vi "S2C_ExeScriptResultCalc.vi"(8 "Error In":errorcluster, 11 "Measurement":string) -> (0 "Error Out":errorcluster, 1 "LastMeas?":bool, 2 "Result":T1, 3 "Data":string[][](array[string]))   [LabVIEW 2015]
doc: "Determines the result for the currently executing line item, and updates the measurement and result in the data array."
uses:
  Controls/S2C_ResultStatus.ctl
  Globals/S2C_Globals.vi
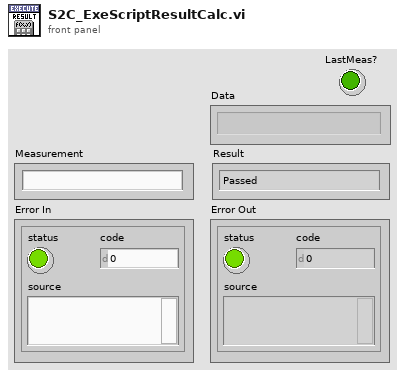
[diagram p1: front panel]
types:
  T1 = typedef "S2C_ResultStatus.ctl" = enum16{"Passed", "Failed", "Logged", "Aborted", "Error", "Testing...", "Paused", "No Record"}
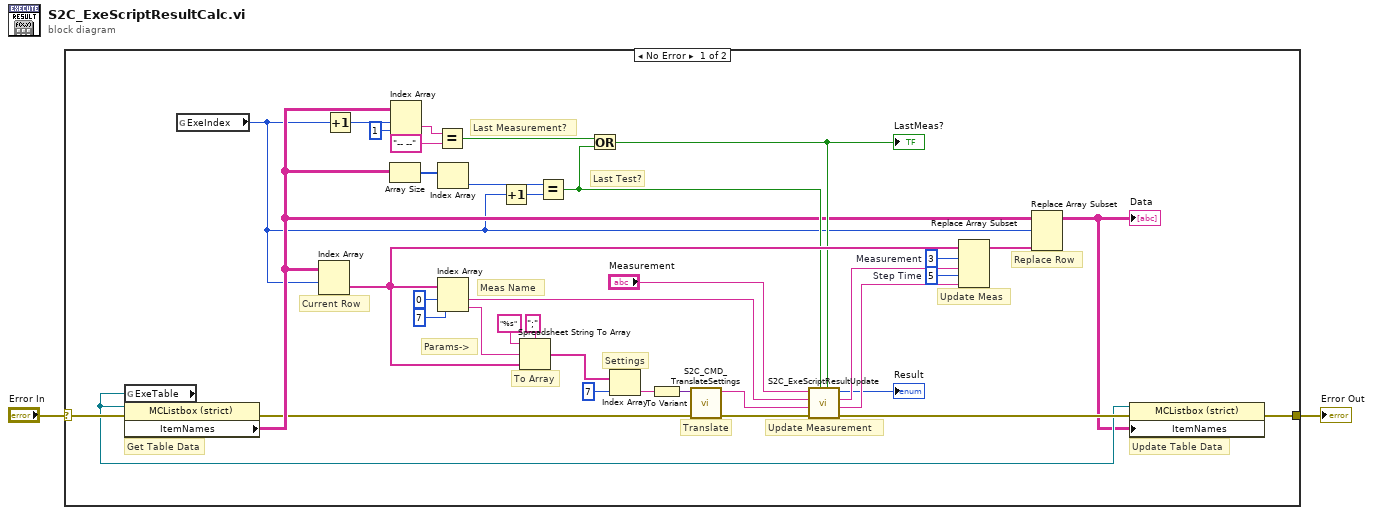
[diagram p0: block diagram]
diagram:
  n1 = case shown="No Error" "Error In" {
    selector: "Error In" -> [w10 w41]
    tunnel: [w4 w41] -> w1
    frame No Error {
      w14 = 5  # Step Time
      w40 = 3  # Measurement
      # "Update Table Data"
      # "Get Table Data"
      # "Last Measurement?"
      # "Update Measurement"
      # "Params->"
      # "To Array"
      # "Translate"
      # "Settings"
      # "Meas Name"
      # "Last Test?"
      # "Replace Row"
      # "Update Meas"
      # "Current Row"
      n2 = global read "S2C_Globals.vi" "ExeTable"() -> (w5:refnum<vi>)
      n3 = property class="MCListbox (strict)"(reference=w5, error in=w10) -> (error out=w8:errorcluster, "ItemNames"=w9:string[][])  [unwired: 1 out]
      n4 = global read "S2C_Globals.vi" "ExeIndex"() -> (w7:i32)
      n5 = Index Array(array=w9, index (row)=w7) -> (element=w33:string[])  [unwired: 1 in]
      n6 = Increment(x=w7) -> (x+1=w21:i32)
      n7 = Array Size(array=w9) -> (size(s)=w38:i32[])
      n8 = Index Array(array=w9, index (row)=w21, index (col)=1 ("disabled index (col)")) -> (element=w19:string)
      n9 = Equal?(x=w19, y="-- --") -> (x = y?=w16:bool)
      n10 = Index Array(array=w38) -> (element=w22:i32)  [unwired: 1 in]
      n11 = Index Array(array=w33, index #1=0 ("index"), index #2=7 ("index")) -> (element #1=w25:string, element #2=w27:string)
      n12 = Increment(x=w7) -> (x+1=w37:i32)
      n13 = Spreadsheet String To Array(delimiter (Tab)=";", format string="%s", spreadsheet string=w27, array type (2D Dbl)=w33) -> (array=w32:string[])
      n14 = Equal?(x=w22, y=w37) -> (x = y?=w17:bool)
      n15 = Or(x=w16, y=w17) -> (x .or. y?=w11:bool)
      "LastMeas?" <- w11
      n16 = Index Array(array=w32, index=7) -> (element=w29:string)
      n17 = To Variant(anything=w29) -> (Variant=w30:variant)
      n18 = call "S2C_CMD_TranslateSettings.vi"("Error In"=w8, "Data"=w30) -> ("Error Out"=w26:errorcluster, "JSON Cluster"=w24:string)  [unwired: 8 in]
      n19 = call "S2C_ExeScriptResultUpdate.vi"("LastMeas?"=w11, "LastTest?"=w17, "Error In"=w26, "StepSettings"=w24, "MeasName"=w25, "Measurement"="Measurement") -> ("Error Out"=w6:errorcluster, "Time"=w13:string, "MeasOut"=w15:string, "Result"=→"Result":T1)  [unwired: 2 in]
      n20 = Replace Array Subset(array=w33, new element #1=w15, index #1=w40, new element #2=w13, index #2=w14) -> (w39:string[])
      n21 = Replace Array Subset(array=w9, new element=w39, index (row)=w7) -> (w3:string[][])  [unwired: 1 in]
      "Data" <- w3
      n22 = property class="MCListbox (strict)"(reference=w5, error in=w6, "ItemNames"=w3) -> (error out=w4:errorcluster)  [unwired: 1 out]
    }
    frame Error {
    }
  }
  "Error Out" <- w1
